vi "CoerceFrequency.vi"(8 "Fe":dbl=86000000.0, 10 "Frequency IN":dbl=86000000.0) -> (0 "nearest integer value":dbl, 2 "Frequency OUT":dbl)   [LabVIEW 2015]
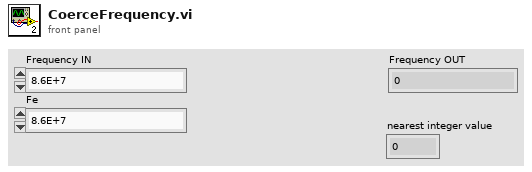
[diagram p1: front panel]
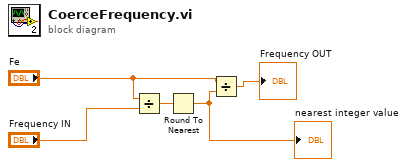
[diagram p0: block diagram]
diagram:
  n1 = Divide(x="Fe", y="Frequency IN") -> (x/y=w4:dbl)
  n2 = Round To Nearest(number=w4) -> (nearest integer value=w3:dbl)
  "nearest integer value" <- w3
  n3 = Divide(x="Fe", y=w3) -> (x/y=→"Frequency OUT":dbl)
